vi "Create Default Wizard Configuration.vi"(8 "error in (no error)":errorcluster, 10 "Reset to default settings? (F)":bool) -> (0 "error out":errorcluster, 3 "Wizard Config Path":path)   [LabVIEW 2018]
uses:
  335fb9bc-462a-45d2-be8a-5357594c188f.vi
  041c5450-aaee-4245-a472-9abb7c78a2bd.vi
  Wizard Strings.vi
  <vilib>/JDP Science/JSONtext/Variant to JSON Text.vi
  <vilib>/JDP Science/JSONtext/JSONtext.lvlib
panel:
  out "Display Text":string
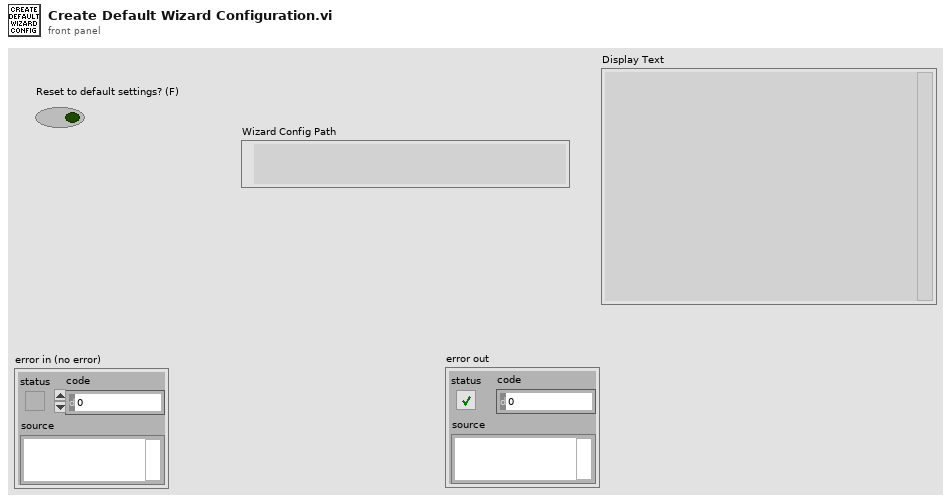
[diagram p1: front panel]
types:
  T1 = enum16{"open", "replace", "create", "open or create", "replace or create", "replace or create with confirmation"}
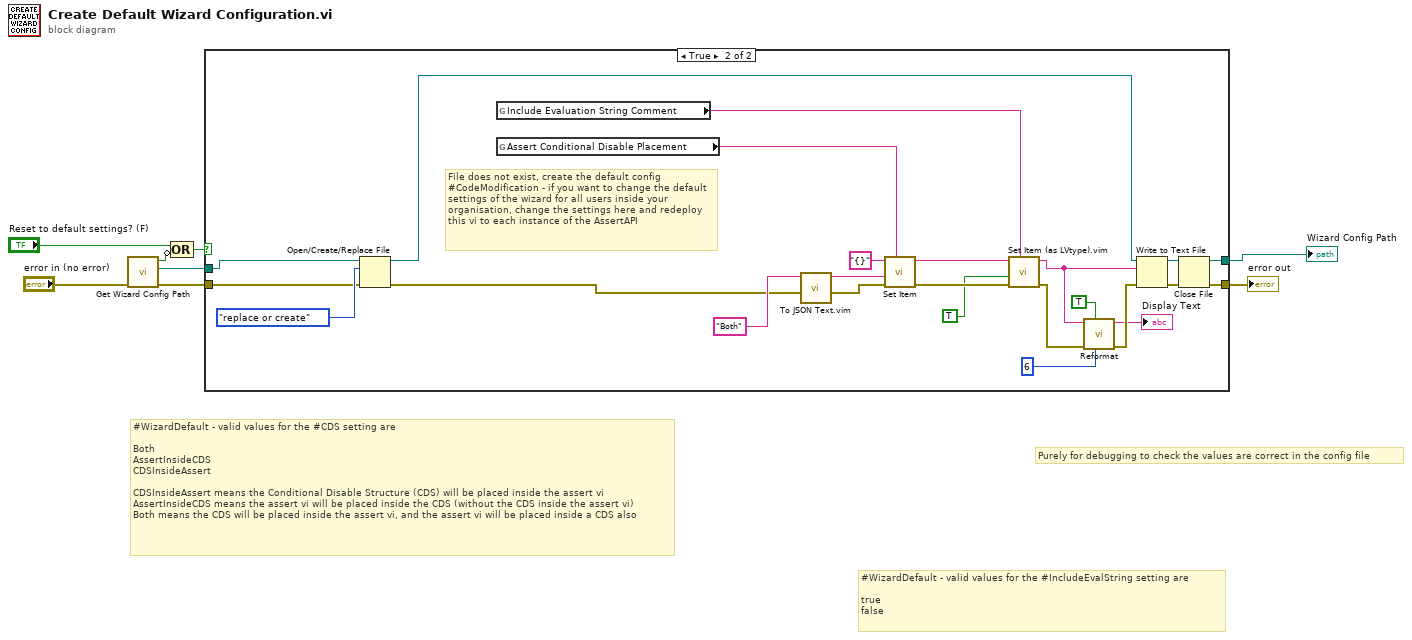
[diagram p0: block diagram]
diagram:
  # "Purely for debugging to check the values are correct in the config file"
  # "#WizardDefault - valid values for the #IncludeEvalString setting are\n\ntrue\nfalse"
  # "#WizardDefault - valid values for the #CDS setting are\n\nBoth\nAssertInsideCDS\nCDSInsideAssert\n\nCDSInsideAssert means the Conditional Disable Structure (CDS) will be placed inside the assert vi\nAssertInsideCDS means the assert vi will be placed inside the CDS (without the CDS inside the assert vi)\nBoth means the CDS will be placed inside the assert vi, and the assert vi will be placed inside a CDS also"
  n1 = call "Get Wizard Config Path.vi"("error in (no error)"="error in (no error)") -> ("error out"=w7:errorcluster, "Wizard Config Path"=w8:path, "Config File Exists"=w3:bool)  [unwired: 8 in]
  n2 = Compound Arithmetic op=OR("Reset to default settings? (F)", invert w3) -> (w1:bool)
  n3 = case shown="True" w1 {
    tunnel: w8 -> [w10 w34]
    tunnel: w7 -> [w9 w32]
    tunnel: [w10 w24] -> w5
    tunnel: [w9 w23] -> w6
    frame False {
      # "File exists - do nothing"
    }
    frame True {
      # "File does not exist, create the default config\n#CodeModification - if you want to change the default settings of the wizard for all users inside your organisation, change the settings here and redeploy this vi to each instance of the AssertAPI"
      n4 = Open/Create/Replace File(file path (use dialog)=w34, error in=w32, operation (0:open)=T1."replace or create") -> (refnum out=w28:refnum<file>, error out=w21:errorcluster)  [unwired: 3 in, 1 out]
      n5 = global read "Wizard Strings.vi" "Include Evaluation String Comment"() -> (w18:string)
      n6 = global read "Wizard Strings.vi" "Assert Conditional Disable Placement"() -> (w19:string)
      n7 = call "To JSON Text.vim"("error in (no error)"=w21, "Anything"="Both" ("$Path or Item Name")) -> ("error out"=w20:errorcluster, "<JSON>"=w30:string)  [unwired: 8 in]
      n8 = call <vilib>:"Set Item.vi"("$Path or Item Name"=w19, "error in (no error)"=w20, "JSON to Insert"=w30, "JSON"="{}") -> ("error out"=w25:errorcluster, "<JSON>"=w22:string)  [unwired: 4 in, 1 out]
      n9 = call "Set Item (as LVtype).vim"("Object (or Item) Path"=w18, "error in (no error)"=w25, "Anything"=TRUE ("Pretty Print?"), "JSON"=w22) -> ("error out"=w17:errorcluster, "<JSON>"=w15:string)  [unwired: 4 in, 1 out]
      n10 = call <vilib>:"Reformat.vi"("Pretty Print Levels"=6, "Alphabetically Sort Objects"=TRUE, "error in (no error)"=w17, "JSON"=w15) -> ("error out"=w16:errorcluster, "<JSON>First JSON Value\n\n<JSON>"=→"Display Text":string)  [unwired: 4 in, 2 out]
      n11 = Write to Text File(file (use dialog)=w28, text=w15, error in=w16) -> (refnum out=w27:refnum<file>, error out=w26:errorcluster)  [unwired: 1 in, 1 out]
      n12 = Close File(refnum=w27, error in=w26) -> (path=w24:path, error out=w23:errorcluster)
    }
  }
  "error out" <- w6
  "Wizard Config Path" <- w5
